vi "Stop Core.vi"(10 "final error code":i32, 11 "Laser_Oxxius in":refnum<class "Laser_Oxxius.lvclass">) -> (3 "Laser_Oxxius out":refnum<class "Laser_Oxxius.lvclass">)   [LabVIEW 2020, in "Laser_Oxxius.lvlib" / "Laser_Oxxius.lvclass"]
doc: "(<B>Filename</B>: Actor Framework.lvlib:Actor.lvclass:Stop Core.vi)\n\nDefines what the actor does before it stops. Use the <B>final error code</B> input to determine whether the actor shut down in response to an error.\n\nBy default, this method passes the Stop message along to all auto-stop nested actors. A descendant class may override this method to define additional behavior, such as shutting down any processes the actor initiated in its override of the Actor Core method."
uses:
  Laser_Oxxius.lvclass
  Laser_Oxxius.lvclass/Laser_Oxxius.ctl
  <vilib>/ActorFramework/Message Enqueuer/Message Enqueuer.lvclass/Message Enqueuer.ctl
  <vilib>/ActorFramework/Message Enqueuer/Enqueue.vi
  <vilib>/ActorFramework/Stop Msg/Stop Msg.lvclass
  C:/Program Files/National Instruments/LabVIEW 2020/vi.lib/ActorFramework/Message/Message.lvclass
  <vilib>/ActorFramework/Message Priority Queue/Priority Enqueue.vi
  HAL Layer/Component/Laser/Laser/Laser.lvclass
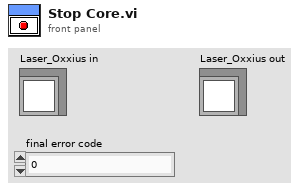
[diagram p1: front panel]
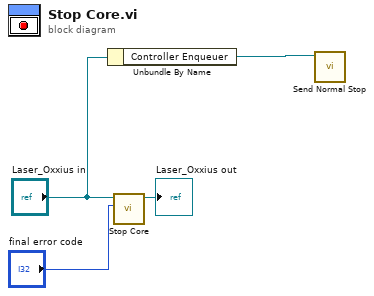
[diagram p0: block diagram]
diagram:
  n1 = Unbundle By Name("Laser_Oxxius in") -> ("Controller Enqueuer"=w2:refnum<class "Message Enqueuer.lvclass">)
  n2 = call-parent "Stop Core.vi"("final error code"="final error code", "Device in"="Laser_Oxxius in") -> ("Device out"=→"Laser_Oxxius out":refnum<class "Laser_Oxxius.lvclass">)  [unwired: 9 in]
  n3 = call <vilib>:"Send Normal Stop.vi"("Message Enqueuer"=w2) -> ()  [unwired: 10 in, 1 out]
